vi "TankFillLevelMaxMinCheck.vi"(9 "max level":dbl, 10 "fill level":dbl, 11 "min level":dbl) -> (1 "below min":bool, 2 "below max":bool, 3 "over min":bool, 4 "over max":bool)   [LabVIEW 2011]
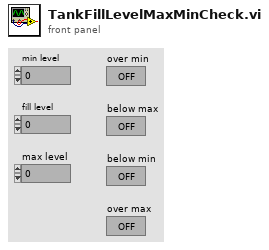
[diagram p1: front panel]
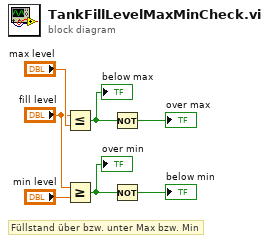
[diagram p0: block diagram]
diagram:
  # "Füllstand über bzw. unter Max bzw. Min"
  n1 = Less Or Equal?(x="fill level", y="max level") -> (x <= y?=w7:bool)
  "below max" <- w7
  n2 = Greater Or Equal?(x="fill level", y="min level") -> (x >= y?=w5:bool)
  "over min" <- w5
  n3 = Not(x=w7) -> (.not. x?=→"over max":bool)
  n4 = Not(x=w5) -> (.not. x?=→"below min":bool)
